vi "Send Start-Stop Message.vi"(6 "Start(T)/Stop(F)":bool, 8 "Error In":errorcluster, 9 "Version number":string, 10 "Software Name":string, 11 "Notebook Queue":refnum<queue>) -> (0 "Error Out":errorcluster)   [LabVIEW 2021, in "Notebook.lvlib"]
uses:
  Notebook.lvlib
  Strings/Strings.lvlib
  Rich Text Box/Text Format List.ctl
  Notebook Action List.ctl
  Notebook Action Q Element.ctl
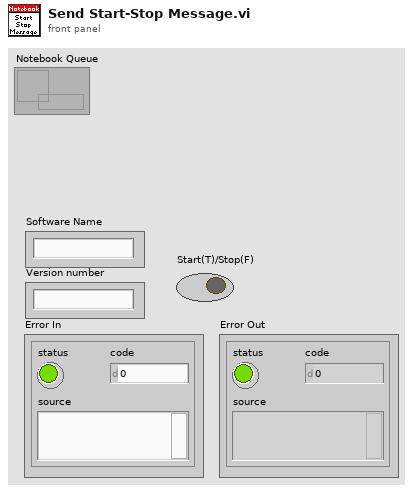
[diagram p1: front panel]
types:
  T1 = typedef "Notebook.lvlib/Text Format List.ctl" = enum16{"Message", "Result", "Error", "Setting", "Verbose", "Warning"}
  T2 = typedef "Rich Text Box.lvlib/Text Formatting.ctl" = cluster{"Font":string, "Text Color":T3, "Background Color":T3, "Style":T4, "Font Size":dbl, "Alignment":T5}
  T3 = typedef "Rich Text Box.lvlib/Text Colors.ctl" = enum16{"Unchanged", "Black", "Blue", "Cyan", "Maroon", "Gray", "Violet", "Green", "Light Green", "Orange", "Yellow", "Magenta", "Red", "White"}
  T4 = typedef "Rich Text Box.lvlib/Text Style.ctl" = enum16{"Regular", "Bold", "Italic", "Underline", "Strikeout"}
  T5 = typedef "Rich Text Box.lvlib/Text Alignment.ctl" = enum16{"Left", "Right", "Center"}
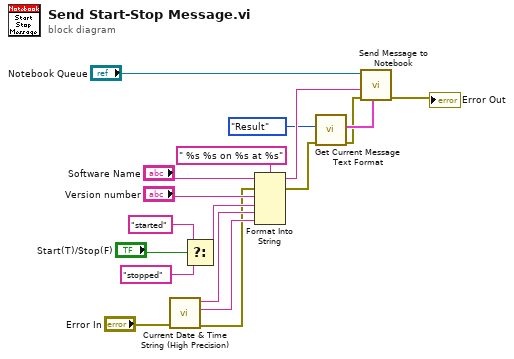
[diagram p0: block diagram]
diagram:
  n1 = call "Current Date & Time String (High Precision).vi"("Error In"="Error In") -> ("Error Out"=w8:errorcluster, "time string"=w11:string, "date string"=w12:string)  [unwired: 7 in, 1 out]
  n2 = Select(t="started" ("Version number"), s="Start(T)/Stop(F)", f="stopped" ("Version number")) -> (s? t:f=w14:string)
  n3 = Format Into String(format string=" %s %s on %s at %s", initial string="Software Name", error in=w8, "Version number", w14, w12, w11) -> (resulting string=w13:string, error out=w2:errorcluster)
  n4 = call "Get Current Message Text Format.vi"("Error In"=w2, "Text Format"=Text_Format_List."Result") -> ("Error Out"=w1:errorcluster, "Message Formatting"=w3:T2)  [unwired: 7 in]
  n5 = call "Send Message to Notebook.vi"("Text Formatting"=w3, "Error In"=w1, "Text"=w13, "Notebook Queue"="Notebook Queue") -> ("Error Out"=→"Error Out":errorcluster)  [unwired: 4 in, 1 out]
